vi "NanoStep ZeroAxis.vi"(0 "VISA Rsrc":refnum<visa-resource-name>="GPIB1::15::INSTR", 5 "Axis":u16(ring)=1 items=["Axis 0", "Axis 1", "All Axis"], 11 "error in":errorcluster) -> (15 "error out":errorcluster)   [LabVIEW 2010]
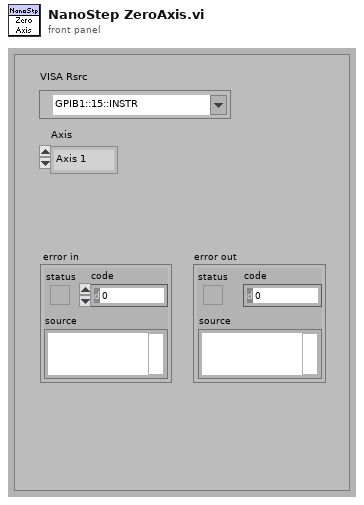
[diagram p1: front panel]
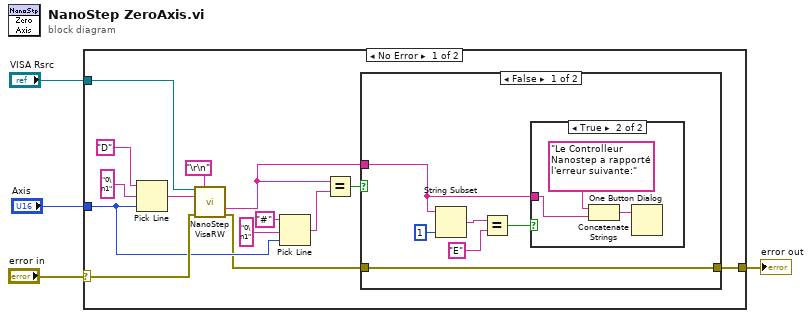
[diagram p0: block diagram]
diagram:
  n1 = case shown="No Error" "error in" {
    selector: "error in" -> [w18 w29]
    tunnel: "Axis" -> [w13 _]
    tunnel: [w8 w29] -> w2
    tunnel: "VISA Rsrc" -> [w17 _]
    frame No Error {
      n2 = Pick Line(string ("")="D" ("chaîne (\"\")"), multi-line string="0\n1" ("x"), line index=w13) -> (output string=w6:string)
      n3 = call <userlib>:"NanoStep VisaRW.vi"("VISA Rsrc"=w17, "EOS (Aucun)"="\r\n", "ChaineCom"=w6, "error in (no error)"=w18) -> ("ChaineRep"=w9:string, "error out"=w7:errorcluster)  [unwired: 8 in, 2 out]
      n4 = Pick Line(string ("")="#" ("chaîne (\"\")"), multi-line string="0\n1" ("x"), line index=w13) -> (output string=w11:string)
      n5 = Equal?(x=w9, y=w11) -> (x = y?=w10:bool)
      n6 = case shown="False" w10 {
        tunnel: w9 -> [w20 _]
        tunnel: [w19 w28] -> w8
        tunnel: w7 -> [w19 w28]
        frame False {
          n7 = String Subset(string=w20, length (rest)=1 ("longueur (reste)")) -> (substring=w21:string)  [unwired: 1 in]
          n8 = Equal?(x=w21, y="E" ("x")) -> (x = y?=w24:bool)
          n9 = case shown="True" w24 {
            tunnel: w20 -> [_ w25]
            frame False {
            }
            frame True {
              n10 = Concatenate Strings("Le Controlleur Nanostep a rapporté l'erreur suivante:", w25) -> (w26:string)
              n11 = One Button Dialog(message=w26) -> ()  [unwired: 1 in, 1 out]
            }
          }
        }
        frame True {
        }
      }
    }
    frame Error {
    }
  }
  "error out" <- w2
